vi "SET_ActiveTool.vi"(8 "error in (no error)":errorcluster, 10 "Radio Buttons":T1, 11 "Tools Paint.lvclass in":refnum<class "Tools Paint.lvclass">) -> (0 "error out":errorcluster, 3 "Tools Paint.lvclass out":refnum<class "Tools Paint.lvclass">)   [LabVIEW 2021, in "Tools Paint.lvclass"]
uses:
  <resource>/plugins/NIIconEditor/Class/Tools/Tools Paint.lvclass
  <resource>/plugins/NIIconEditor/Controls/Tools.ctl
  <resource>/plugins/NIIconEditor/Controls/Pen.ctl
  <resource>/plugins/NIIconEditor/Controls/Line.ctl
  <resource>/plugins/NIIconEditor/Controls/Dropper.ctl
  <resource>/plugins/NIIconEditor/Controls/Fill.ctl
  <resource>/plugins/NIIconEditor/Controls/IERect.ctl
  <resource>/plugins/NIIconEditor/Controls/FRect.ctl
  <resource>/plugins/NIIconEditor/Controls/Circle.ctl
  <resource>/plugins/NIIconEditor/Controls/FCircle.ctl
  <resource>/plugins/NIIconEditor/Controls/Rubber.ctl
  <resource>/plugins/NIIconEditor/Controls/Text.ctl
  <resource>/plugins/NIIconEditor/Controls/Selection.ctl
  <resource>/plugins/NIIconEditor/Controls/Move.ctl
  <resource>/plugins/NIIconEditor/Class/Tools/Tools Paint.lvclass/Tools Paint.ctl
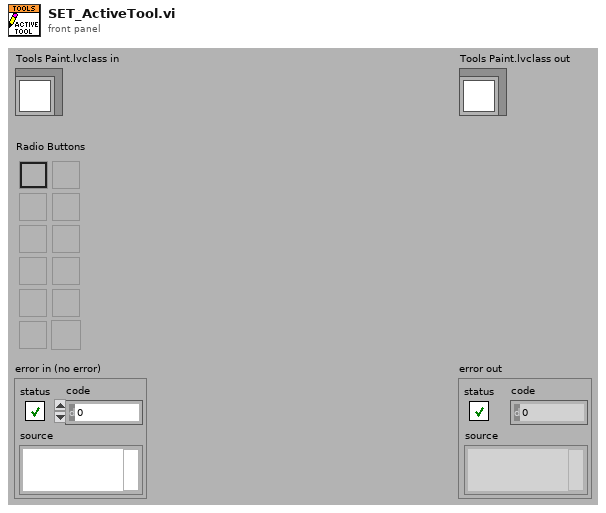
[diagram p1: front panel]
types:
  T1 = typedef "Tools.ctl" = enum32{"Pencil", "Line", "Dropper", "Fill", "Rectangle", "Filled Rectangle", "Ellipse", "Filled Ellipse", "Eraser", "Text", "Select", "Move"}
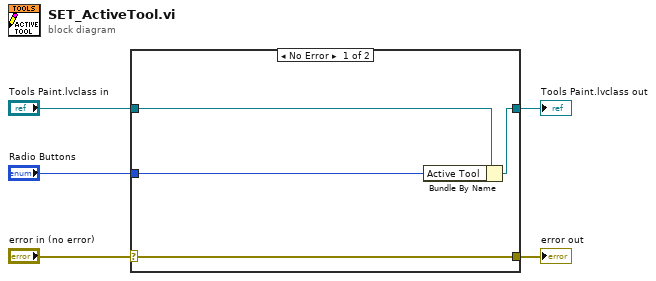
[diagram p0: block diagram]
diagram:
  n1 = case shown="No Error" "error in (no error)" {
    selector: "error in (no error)" -> [w9 w10]
    tunnel: [w9 w10] -> w4
    tunnel: [w7 w11] -> w2
    tunnel: "Tools Paint.lvclass in" -> [w8 w11]
    tunnel: "Radio Buttons" -> [w6 _]
    frame No Error {
      n2 = Bundle By Name(cluster=w8, "Active Tool"=w6) -> (w7:refnum<class "Tools Paint.lvclass">)
    }
    frame Error {
    }
  }
  "error out" <- w4
  "Tools Paint.lvclass out" <- w2
